vi "Get All Test Registrations.vi"(8 "error in (no error)":errorcluster, 11 "Test Event Storage in":refnum<class "Test Event Storage.lvclass">) -> (0 "error out":errorcluster, 1 "Test Registrations":T1[](array[typedef]), 2 "Keys":string[](array[string]), 3 "Test Event Storage out":refnum<class "Test Event Storage.lvclass">, 5 "Parent Keys":string[](array[string]))   [LabVIEW 2009, in "Caraya.lvlib" / "Test Event Storage.lvclass"]
uses:
  Test Event Storage.lvclass
  Test Result/Test Node.ctl
  Test Result/Test Registration Data.ctl
  Test Event Storage.lvclass/Test Event Storage.ctl
  Test Result/Test Result.lvclass
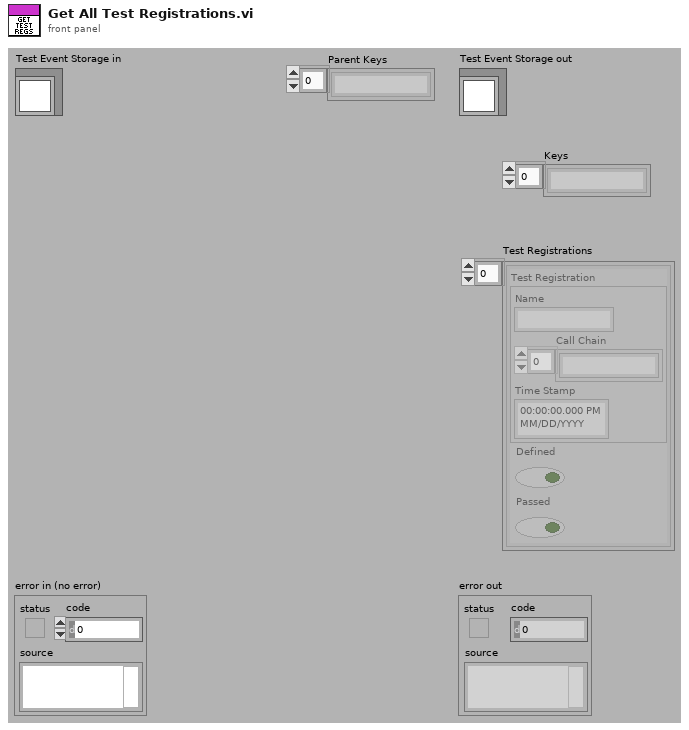
[diagram p1: front panel]
types:
  T1 = typedef "Caraya.lvlib/Test Result.lvclass/Test Node.ctl" = cluster{"Test Registration":T2, "Defined":bool, "Passed":bool}
  T2 = typedef "Caraya.lvlib/Test Result.lvclass/Test Registration Data.ctl" = cluster{"Name":string, "Call Chain":string[], "Time Stamp":timestamp}
  T3 = cluster{i32, "Key":string, "Key":string, "Test Node":T1}
  T4 = cluster{i32, "Key":string, "Key":string, "Test Node":T1}[]
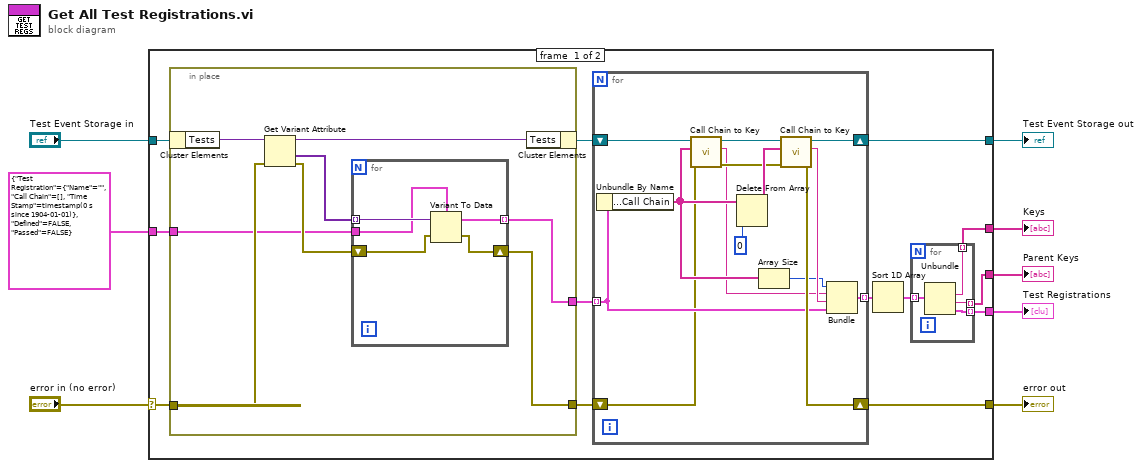
[diagram p0: block diagram]
diagram:
  n1 = case shown="No Error" "error in (no error)" {
    selector: "error in (no error)" -> [w20 w54]
    tunnel: [w14 w54] -> w7
    tunnel: [w17 w53] -> w5
    tunnel: "Test Event Storage in" -> [w21 w53]
    tunnel: T1 {"Test Registration"={"Name"="", "Call Chain"=[], "Time Stamp"=timestamp(0 s since 1904-01-01)}, "Defined"=FALSE, "Passed"=FALSE} ("Test Node") -> [w19 _]
    tunnel: [w11 _] -> w4
    tunnel: [w10 _] -> w2
    tunnel: [w9 _] -> w1
    frame #0 {
      n2 = in-place {
        in-place-border: w20 -> [w46]
        in-place-border: [w42] -> w15
        in-place-border: w19 -> [w41]
        in-place-border: [w40] -> w16
        n3 = in-place-cluster #1(w21) -> ("Tests"=w47:variant)
        n4 = Get Variant Attribute(Variant=w47, error in=w46) -> (duplicate Variant=w45:variant, values=w44:variant[], error out=w43:errorcluster)  [unwired: 2 in, 1 out]
        n5 = for {
          tunnel: w44 -> [w52] mode=indexing
          tunnel: w41 -> [w51]
          shift-right: [w49] -> w42
          shift-left: w43 -> [w50]
          tunnel: [w48] -> w40 mode=indexing
          n6 = Variant To Data(error in=w50, Variant=w52, type=w51) -> (error out=w49:errorcluster, data=w48:T1)
        }
        n7 = in-place-cluster #1("Tests"=w45) -> (w18:refnum<class "Test Event Storage.lvclass">)
      }
      n8 = for {
        shift-right: [w39] -> w17
        shift-left: w18 -> [w32]
        tunnel: w16 -> [w33] mode=indexing
        shift-right: [w36] -> w14
        shift-left: w15 -> [w28]
        tunnel: [w35] -> w13 mode=indexing
        n9 = Unbundle By Name(w33) -> ("Test Registration.Call Chain"=w29:string[])
        n10 = call "Call Chain to Key.vi"("error in (no error)"=w28, "Call Chain"=w29, "Test Event Storage in"=w32) -> ("error out"=w30:errorcluster, "Key"=w26:string, "Test Event Storage out"=w31:refnum<class "Test Event Storage.lvclass">)  [unwired: 6 in]
        n11 = Delete From Array(array=w29, index=0) -> (array with subset deleted=w37:string[])  [unwired: 1 in, 1 out]
        n12 = Array Size(array=w29) -> (size(s)=w27:i32)
        n13 = call "Call Chain to Key.vi"("error in (no error)"=w30, "Call Chain"=w37, "Test Event Storage in"=w31) -> ("error out"=w36:errorcluster, "Key"=w34:string, "Test Event Storage out"=w39:refnum<class "Test Event Storage.lvclass">)  [unwired: 6 in]
        n14 = Bundle(w27, "Key"=w26, "Key"=w34, "Test Node"=w33) -> (w35:T3)  [unwired: 1 in]
      }
      n15 = Sort 1D Array(array=w13) -> (sorted array=w12:T4)
      n16 = for {
        tunnel: w12 -> [w25] mode=indexing
        tunnel: [w24] -> w11 mode=indexing
        tunnel: [w22] -> w10 mode=indexing
        tunnel: [w23] -> w9 mode=indexing
        n17 = Unbundle(w25) -> ("Key"=w23:string, "Key"=w22:string, "Test Node"=w24:T1)  [unwired: 1 out]
      }
    }
    frame #1 {
    }
  }
  "error out" <- w7
  "Test Event Storage out" <- w5
  "Test Registrations" <- w4
  "Parent Keys" <- w2
  "Keys" <- w1
